vi "Pic with Tube_0.1 (SubVI).vi"() -> (3 "Picture":i32[][](array[numeric]))   [LabVIEW 2013]
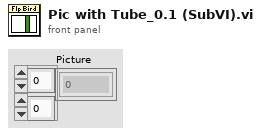
[diagram p1: front panel]
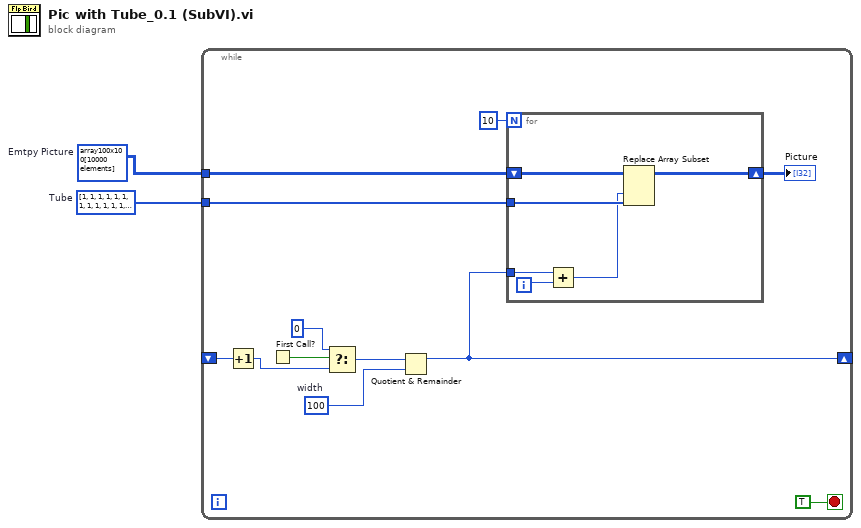
[diagram p0: block diagram]
diagram:
  w1 = i32[] [1, 1, 1, 1, 1, 1, 1, 1, 1, 1, 1, 1, 1, 1, 1, 1, 1, 1, 1, 1, 1, 1, 1, 1, 1, 1, 1, 1, 1, 1, 1, 1, 1, 1, 1, 1, 1, 1, 1, 1, 1, 1, 1, 1, 1, 1, 1, 1, 1, 1, 1, 1, 1, 1, 1, 1, 1, 1, 1, 1, 1, 1, 1, 1, 1, 1, 1, 1, 1, 1, 1, 1, 1, 1, 1, 1, 1, 1, 1, 1, 1, 1, 1, 1, 1, 1, 1, 1, 1, 1, 1, 1, 1, 1, 1, 1, 1, 1, 1, 1]  # Tube
  w2 = i32[][] array100x100[10000 elements]  # Emtpy Picture
  n1 = while {
    shift-right: [w6] -> _
    shift-left: _ -> [w12]
    tunnel: w2 -> [w4]
    tunnel: w1 -> [w3]
    stop <- TRUE stop-if-true
    w9 = 100  # width
    n2 = Increment(x=w12) -> (x+1=w11:i32)
    n3 = First Call?() -> (First Call?: T/F=w10:bool)
    n4 = Select(t=0, s=w10, f=w11) -> (s? t:f=w13:i32)
    n5 = Quotient & Remainder(x=w13, y=w9) -> (x-y*floor(x/y)=w6:i32)  [unwired: 1 out]
    n6 = for {
      N: 10 -> [_]
      shift-right: [w19] -> w8
      shift-left: w4 -> [w20]
      tunnel: w6 -> [w17]
      tunnel: w3 -> [w16]
      i -> [w18]
      n7 = Add(x=w17, y=w18) -> (x+y=w15:i32)
      n8 = Replace Array Subset(array=w20, new element=w16, index (col)=w15) -> (w19:i32[][])  [unwired: 1 in]
    }
    "Picture" <- w8
  }
